vi "main.vi"() -> ()   [LabVIEW 2024]
uses:
  C:/Users/QLM-CCD/Desktop/Pump probe/Kinesis/Thorlabs.MotionControl.Benchtop.BrushlessMotorCLI.dll
  Kinesis/Thorlabs.MotionControl.Benchtop.BrushlessMotorCLI.dll
  <vilib>/Utility/file.llb/Read Delimited Spreadsheet (DBL).vi
  <vilib>/Utility/file.llb/Write Delimited Spreadsheet (DBL).vi
  C:/Users/QLM-CCD/Desktop/Pump probe/Kinesis/Thorlabs.MotionControl.Controls.dll
  Kinesis/Thorlabs.MotionControl.Controls.dll
  <instrlib>/Thorlabs_MC2000B/Thorlabs_MC2000B.lvlib
panel:
  out "return value":string[](array[string])
  out "pp_sig_avg":dbl[](array[numeric])
  out "pp_sig_sum":dbl[](array[numeric])
  in  "Tab Control":enum32{"main", "advanced", "documents"}(tab)
  out "is_measure":bool
  in  "measure_rounds":i16=1 caption="X"
  out "current_delay":dbl caption="fs" format="%#_5g"
  in  "stop":bool
  out "pump probe signal cont":dbl(graph)
  in  "Save_data_path":path=path "C:/Users/QLM-CCD/Desktop/Pump probe/test/test.txt"
  out "XY Graph":cluster{"Y":dbl[], "Y":dbl[]}[](graph)
  out "measure_progress":u8(slide) scale=0.0..12.0
  in  "measure":bool
  in  "Set zero":bool
  in  "measure_cont":bool
  out "is_measure_cont":bool
  in  "delay_profile":u16(ring) caption="delay profile" items=["test", "test2", "test3"]
  in  "set delay":dbl caption="move"
  in  "Set frequency (Hz)":i32=1000
  out "Chopper Frequency (Hz)":i32 caption="chopper freq."
  in  "set lock-in Integration time":dbl=100.0 caption="integration time"
  in  "delay list":dbl[](array[numeric])
  in  "device position (mm)":dbl
  out "Lock-in Integration time":dbl caption="integration time"
  in  "BenchtopBrushlessControl":refnum<k24>(container)
  in  "stop 2":bool
  in  "save_profile":bool
  in  "profile_name":string caption="delay profile"
  in  "open_doc_SR830":bool
  in  "open_doc_MC2000B":bool
  in  "open_doc_BBD301":bool
  out "pp_sig_sgl":dbl[](array[numeric])
  # "todo: state machine,\nfs-ps switch,, note box, issue report box, change color when delay stage is moveing,  measure background, hide kinesis panel"
  # "#BUG: Start measurement without save file will crash"
  # "pump probe  ver0.1.1  2024.08.02"
  # "Hz"
  # "Hz"
  # "ms"
  # "ms"
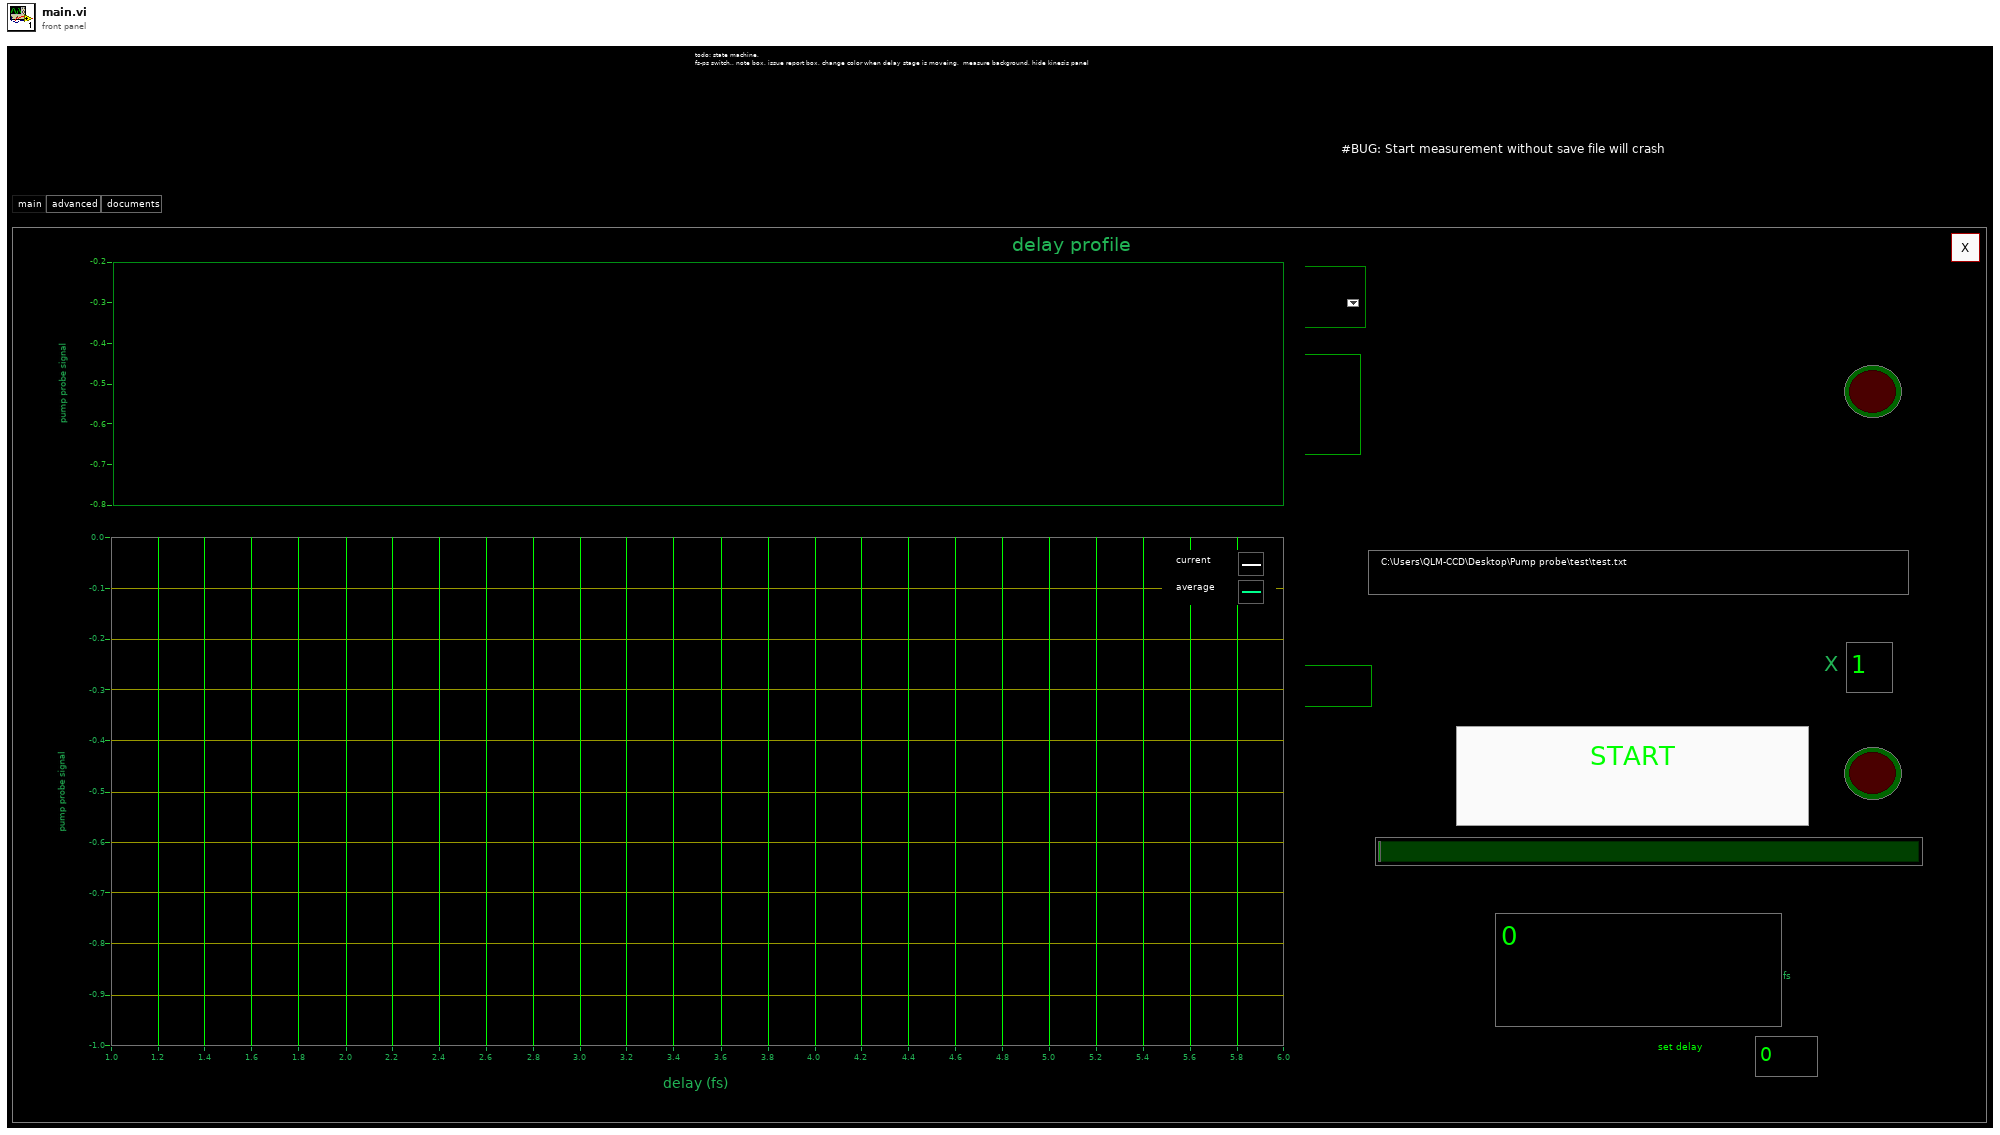
[diagram p1: front panel]
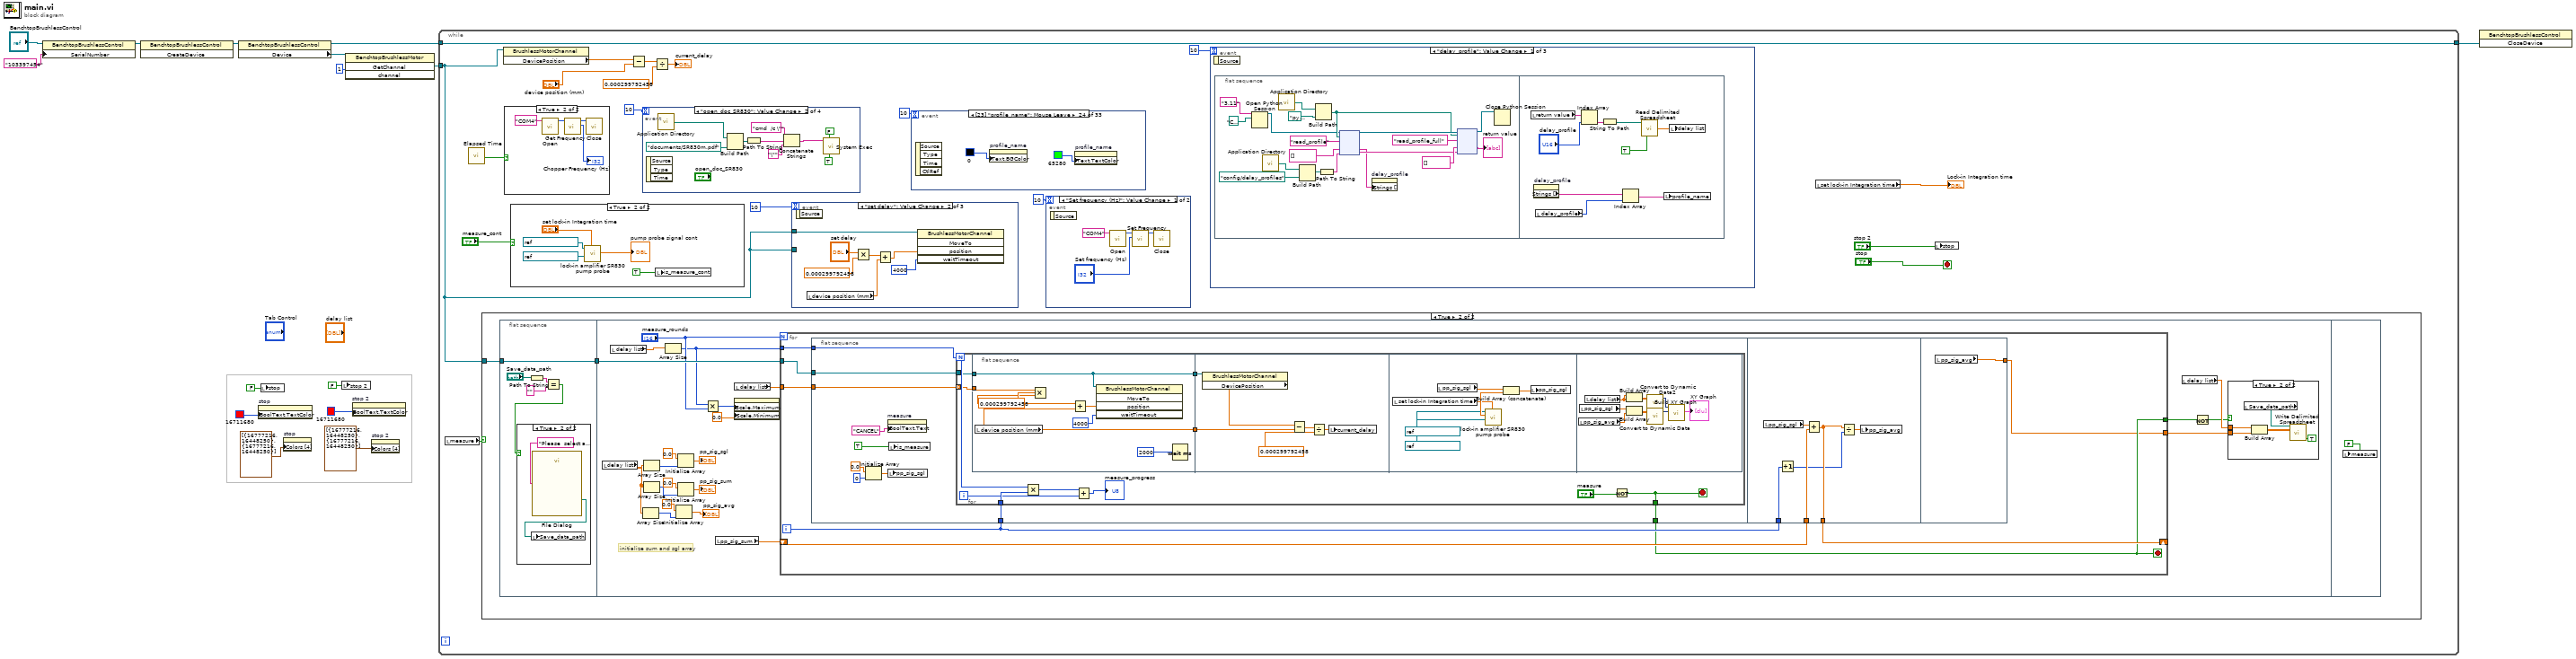
[diagram p0: block diagram]
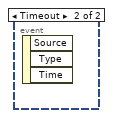
[diagram p2: hidden frame]
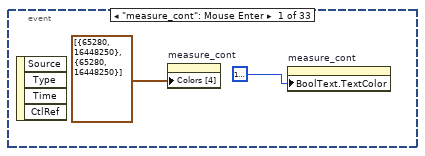
[diagram p3: hidden frame]
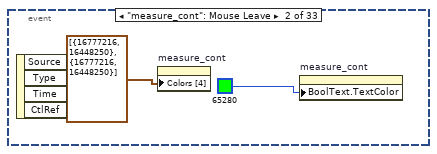
[diagram p4: hidden frame]
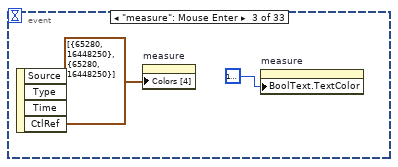
[diagram p5: hidden frame]
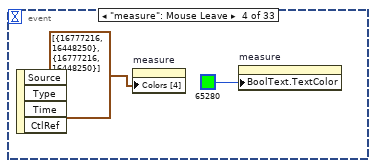
[diagram p6: hidden frame]
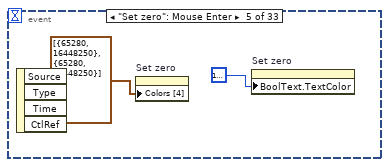
[diagram p7: hidden frame]
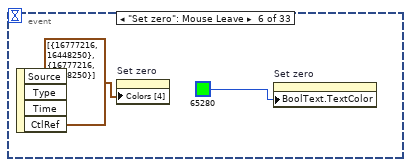
[diagram p8: hidden frame]
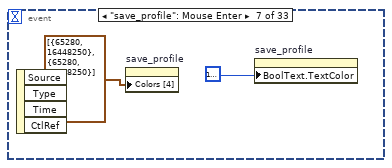
[diagram p9: hidden frame]
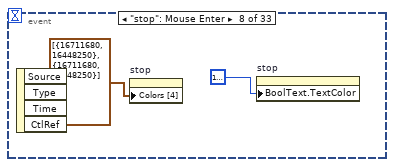
[diagram p10: hidden frame]
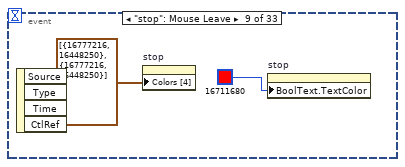
[diagram p11: hidden frame]
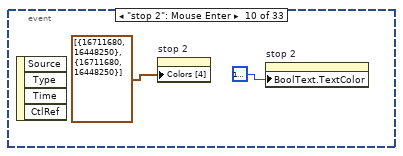
[diagram p12: hidden frame]
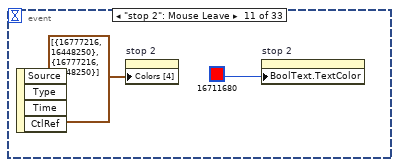
[diagram p13: hidden frame]
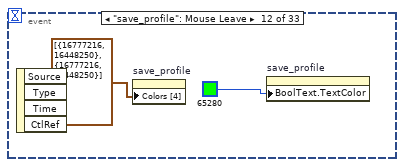
[diagram p14: hidden frame]
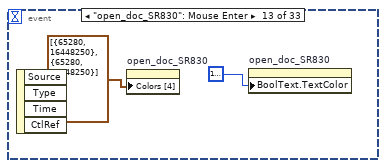
[diagram p15: hidden frame]
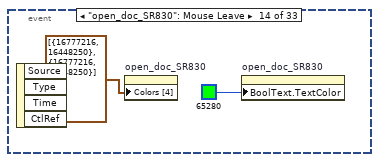
[diagram p16: hidden frame]
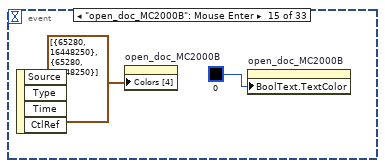
[diagram p17: hidden frame]
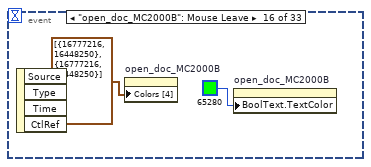
[diagram p18: hidden frame]
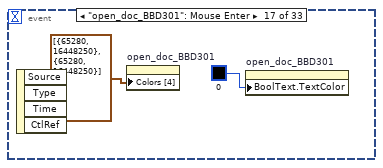
[diagram p19: hidden frame]
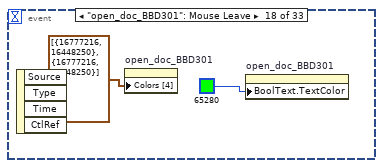
[diagram p20: hidden frame]
diagram:
  n1 = property class="BenchtopBrushlessControl"(reference="BenchtopBrushlessControl", "SerialNumber"="103397454") -> (reference out=w14:refnum<k24>)  [unwired: 1 in, 1 out]
  n2 = invoke class="BenchtopBrushlessControl" method="CreateDevice"(reference=w14) -> (reference out=w13:refnum<k24>)  [unwired: 2 in, 2 out]
  n3 = property class="BenchtopBrushlessControl"(reference=w13) -> (reference out=w11:refnum<k24>, "Device"=w5:refnum<k24>)  [unwired: 1 in, 1 out]
  n4 = property on="stop" class="Bool (strict)"("BoolText.TextColor"=u32 16711680) -> ()  [unwired: 2 in, 2 out]
  n5 = local write "stop"(FALSE ("is_measure")) -> ()
  n6 = property on="stop" class="Bool (strict)"("Colors [4]"=cluster{u32, u32}[] [{16777216, 16448250}, {16777216, 16448250}]) -> ()  [unwired: 2 in, 2 out]
  n7 = local write "stop 2"(FALSE ("is_measure")) -> ()
  n8 = invoke class="BenchtopBrushlessMotor" method="GetChannel"(reference=w5, "channel"=i16 1) -> ("GetChannel"=w8:refnum<k24>)  [unwired: 2 in, 3 out]
  n9 = property on="stop 2" class="Bool (strict)"("BoolText.TextColor"=u32 16711680) -> ()  [unwired: 2 in, 2 out]
  n10 = property on="stop 2" class="Bool (strict)"("Colors [4]"=cluster{u32, u32}[] [{16777216, 16448250}, {16777216, 16448250}]) -> ()  [unwired: 2 in, 2 out]
  n11 = while {
    tunnel: w11 -> [w33]
    tunnel: [w33] -> w10
    tunnel: w8 -> [w16]
    stop <- "stop" stop-if-true
    n12 = local read "measure"() -> (w22:bool)
    n13 = call "Elapsed Time"() -> ("Time has Elapsed"=w27:bool)  [unwired: 12 in, 7 out]
    n14 = case shown="True" w22 {
      tunnel: w16 -> [_ w106]
      frame False {
        n15 = local write "measure_progress"(u8 0 ("measure_progress")) -> ()
        n16 = property on="measure" class="Bool (strict)"("BoolText.Text"="START" ("Boolean Text.Text")) -> ()  [unwired: 2 in, 2 out]
        "is_measure" <- FALSE ("is_measure")
      }
      frame True {
        n17 = flat-sequence {
          tunnel: w106 -> [w111]
          tunnel: [w111] -> w105
          tunnel: w105 -> [w125]
          frame #0 {
            n18 = Path To String(path="Save_data_path") -> (string=w110:string)
            n19 = Equal?(x=w110, y="") -> (x = y?=w107:bool)
            n20 = case shown="True" w107 {
              frame False {
              }
              frame True {
                n21 = call "File Dialog"("prompt"="Please  select a file to save your data") -> ("selected path"=w112:path)  [unwired: 11 in, 3 out]
                n22 = local write "Save_data_path"(w112) -> ()
              }
            }
          }
          frame #1 {
            # "initialize sum and sgl array"
            n23 = local read "delay list"() -> (w122:dbl[])
            n24 = local read "delay list"() -> (w134:dbl[])
            n25 = Array Size(array=w122) -> (size(s)=w123:i32)
            n26 = Array Size(array=w122) -> (size(s)=w131:i32)
            n27 = Array Size(array=w122) -> (size(s)=w129:i32)
            n28 = Array Size(array=w134) -> (size(s)=w116:i32)
            n29 = Initialize Array(0.0 ("element"), w123) -> (→"pp_sig_avg":dbl[])
            n30 = Initialize Array(0.0 ("element"), w131) -> (→"pp_sig_sgl":dbl[])
            n31 = Initialize Array(0.0 ("element"), w129) -> (→"pp_sig_sum":dbl[])
            n32 = Multiply(x=w116, y="measure_rounds") -> (x*y=w135:i32)
            n33 = local read "pp_sig_sum"() -> (w128:dbl[])
            n34 = local read "delay list"() -> (w118:dbl[])
            n35 = property on="measure_progress" class="Slide (strict)"("Scale.Maximum"=w135, "Scale.Minimum"=0.0 ("Scale.Range:Minimum")) -> ()  [unwired: 2 in, 2 out]
            n36 = for {
              N: "measure_rounds" -> [_]
              tunnel: w125 -> [w138]
              shift-right: [w143] -> _
              shift-left: w128 -> [w142]
              tunnel: w118 -> [w140]
              tunnel: [w139] -> w117
              tunnel: w116 -> [w137]
              tunnel: [w136] -> w114
              i -> [w141]
              stop <- w139 stop-if-true
              n37 = flat-sequence {
                tunnel: w141 -> [w153]
                tunnel: [w152] -> w139
                tunnel: w140 -> [w151]
                tunnel: w138 -> [w148]
                tunnel: w137 -> [w147]
                tunnel: w141 -> [w194]
                tunnel: [w197] -> w143
                tunnel: w142 -> [w196]
                tunnel: [w199] -> w136
                frame #0 {
                  n38 = Initialize Array(0.0 ("element"), 0 ("dimension size")) -> (w146:dbl[])
                  n39 = property on="measure" class="Bool (strict)"("BoolText.Text"="CANCEL" ("Boolean Text.Text")) -> ()  [unwired: 2 in, 2 out]
                  n40 = local write "pp_sig_sgl"(w146) -> ()
                  n41 = local write "is_measure"(TRUE ("is_measure")) -> ()
                  n42 = for {
                    N: w147 -> [w160]
                    tunnel: [w159] -> w152
                    tunnel: w153 -> [w161]
                    tunnel: w151 -> [w156] mode=indexing
                    tunnel: w148 -> [w155]
                    i -> [w157]
                    stop <- w159 stop-if-true
                    n43 = flat-sequence {
                      tunnel: [w169] -> w164
                      tunnel: w156 -> [w167]
                      tunnel: w155 -> [w165]
                      tunnel: [w165] -> w154
                      tunnel: w164 -> [w177]
                      tunnel: w154 -> [w173]
                      frame #0 {
                        n44 = local read "device position (mm)"() -> (w169:dbl)
                        n45 = Multiply(x=w167, y=0.000299792458) -> (x*y=w172:dbl)
                        n46 = Add(x=w172, y=w169) -> (x+y=w170:dbl)
                        n47 = invoke class="BrushlessMotorChannel" method="MoveTo"(reference=w165, "position"=w170, "waitTimeout"=4000) -> ()  [unwired: 2 in, 5 out]
                        n48 = Wait (ms)(milliseconds to wait=u32 2000) -> ()  [unwired: 1 out]
                      }
                      frame #1 {
                        n49 = property class="BrushlessMotorChannel"(reference=w173) -> ("DevicePosition"=w174:dbl)  [unwired: 1 in, 2 out]
                        n50 = Subtract(x=w174, y=w177) -> (x-y=w178:dbl)
                        n51 = Divide(x=w178, y=0.000299792458) -> (x/y=w176:dbl)
                        n52 = local write "current_delay"(w176) -> ()
                      }
                      frame #2 {
                        n53 = local read "set lock-in Integration time"() -> (w181:dbl)
                        n54 = local read "pp_sig_sgl"() -> (w180:dbl[])
                        n55 = call "lock-in amplifier SR830 pump probe.vi"("Integration time (ms)"=w181, "Connection 2"=refnum<visa-resource-name> "GPIB0::5::INSTR", "Connection"=refnum<visa-resource-name> "GPIB1::2::INSTR") -> ("pump probe signal"=w183:dbl)  [unwired: 8 in]
                        n56 = Build Array (concatenate)(w180, w183) -> (w179:dbl[])
                        n57 = local write "pp_sig_sgl"(w179) -> ()
                      }
                      frame #3 {
                        n58 = local read "pp_sig_avg"() -> (w187:dbl[])
                        n59 = local read "pp_sig_sgl"() -> (w185:dbl[])
                        n60 = local read "delay list"() -> (w190:dbl[])
                        n61 = Build Array(w190, w190) -> (w189:dbl[][])
                        n62 = Build Array(w185, w187) -> (w191:dbl[][])
                        n63 = call "Convert to Dynamic Data2"("2D Array"=w189) -> ("Dynamic Data Type"=w188:dynamicdata)  [unwired: 3 in]
                        n64 = call "Convert to Dynamic Data"("2D Array"=w191) -> ("Dynamic Data Type"=w192:dynamicdata)  [unwired: 3 in]
                        n65 = call "Build XY Graph"("Y Input"=w192, "X Input"=w188) -> ("XY Graph"=→"XY Graph":cluster{"X":dbl[], "Y":dbl[]}[])  [unwired: 8 in, 1 out]
                      }
                    }
                    n66 = Multiply(x=w160, y=w161) -> (x*y=w158:i32)
                    n67 = Add(x=w158, y=w157) -> (x+y=→"measure_progress":i32)
                    n68 = Not(x="measure") -> (.not. x?=w159:bool)
                  }
                }
                frame #1 {
                  n69 = local read "pp_sig_sgl"() -> (w198:dbl[])
                  n70 = Increment(x=w194) -> (x+1=w193:i32)
                  n71 = Add(x=w198, y=w196) -> (x+y=w197:dbl[])
                  n72 = Divide(x=w197, y=w193) -> (x/y=w195:dbl[])
                  n73 = local write "pp_sig_avg"(w195) -> ()
                }
                frame #2 {
                  n74 = local read "pp_sig_avg"() -> (w199:dbl[])
                }
              }
            }
            n75 = local read "delay list"() -> (w133:dbl[])
            n76 = Not(x=w117) -> (.not. x?=w115:bool)
            n77 = case shown="True" w115 {
              tunnel: w133 -> [_ w202]
              tunnel: w114 -> [_ w200]
              frame False {
              }
              frame True {
                n78 = local read "Save_data_path"() -> (w201:path)
                n79 = Build Array(w202, w200) -> (w204:dbl[][])
                n80 = call-poly <vilib>:"Write Delimited Spreadsheet.vi"("file path (dialog if empty)"=w201, "2D data"=w204, "transpose? (no:F)"=TRUE) -> ()  [unwired: 11 in, 2 out]
              }
            }
          }
          frame #2 {
            n81 = local write "measure"(FALSE ("measure")) -> ()
          }
        }
      }
    }
    n82 = property class="BrushlessMotorChannel"(reference=w16) -> ("DevicePosition"=w31:dbl)  [unwired: 1 in, 2 out]
    n83 = case shown="True" w27 {
      frame False {
      }
      frame True {
        n84 = call <instrlib>:"Open.vi"("Serial Port"="COM4") -> ("Handle out"=w278:i32)  [unwired: 8 in, 2 out]
        n85 = call <instrlib>:"Get Frequency.vi"("Handle in"=w278) -> ("Frequency (Hz)"=→"Chopper Frequency (Hz)":i32, "Handle out"=w277:i32)  [unwired: 8 in, 1 out]
        n86 = call <instrlib>:"Close.vi"("hdl"=w277) -> ()  [unwired: 10 in, 1 out]
      }
    }
    n87 = case shown="True" "measure_cont" {
      frame False {
        "is_measure_cont" <- FALSE ("is_measure_cont")
      }
      frame True {
        n88 = call "lock-in amplifier SR830 pump probe.vi"("Integration time (ms)"="set lock-in Integration time", "Connection 2"=refnum<visa-resource-name> "GPIB0::5::INSTR", "Connection"=refnum<visa-resource-name> "GPIB1::2::INSTR") -> ("pump probe signal"=→"pump probe signal cont":dbl)  [unwired: 8 in]
        n89 = local write "is_measure_cont"(TRUE ("is_measure_cont")) -> ()
      }
    }
    n90 = Subtract(x=w31, y="device position (mm)") -> (x-y=w30:dbl)
    n91 = event shown="[1] \"open_doc_SR830\": Value Change" {
      selector: _ -> [_ _ _ _]
      dyn-events: _ -> [_ _ _ _]
      timeout: 10 -> [_ _ _ _]
      event Timeout {
        n92 = event-data() -> ()  [unwired: 1 in, 3 out]
      }
      event "open_doc_SR830": Value Change {
        n93 = event-data() -> ()  [unwired: 1 in, 3 out]
        n94 = call <vilib>:"Application Directory.vi"() -> ("Application Directory"=w245:path)
        n95 = Build Path(base path=w245, name or relative path=path "documents/SR830m.pdf") -> (appended path=w246:path)
        n96 = Path To String(path=w246) -> (string=w244:string)
        n97 = Concatenate Strings("cmd  /c \"" ("string"), w244, "\"" ("string")) -> (w250:string)
        n98 = call <vilib>:"System Exec.vi"("run minimized? (F)"=TRUE, "wait until completion? (T)"=FALSE, "command line"=w250) -> ()  [unwired: 5 in, 4 out]
      }
      event "open_doc_MC2000B": Value Change {
        n99 = event-data() -> ()  [unwired: 1 in, 3 out]
        n100 = call <vilib>:"Application Directory.vi"() -> ("Application Directory"=w254:path)
        n101 = Build Path(base path=w254, name or relative path=path "documents/MC2000B-Manual.pdf") -> (appended path=w255:path)
        n102 = Path To String(path=w255) -> (string=w252:string)
        n103 = Concatenate Strings("cmd  /c \"" ("string"), w252, "\"" ("string")) -> (w259:string)
        n104 = call <vilib>:"System Exec.vi"("run minimized? (F)"=TRUE, "wait until completion? (T)"=FALSE, "command line"=w259) -> ()  [unwired: 5 in, 4 out]
      }
      event "open_doc_BBD301": Value Change {
        n105 = event-data() -> ()  [unwired: 1 in, 1 out]
        n106 = call <vilib>:"Application Directory.vi"() -> ("Application Directory"=w263:path)
        n107 = Build Path(base path=w263, name or relative path=path "documents/BBD301-KinesisManual.pdf") -> (appended path=w264:path)
        n108 = Path To String(path=w264) -> (string=w261:string)
        n109 = Concatenate Strings("cmd  /c \"" ("string"), w261, "\"" ("string")) -> (w268:string)
        n110 = call <vilib>:"System Exec.vi"("run minimized? (F)"=TRUE, "wait until completion? (T)"=FALSE, "command line"=w268) -> ()  [unwired: 5 in, 4 out]
      }
    }
    n111 = Divide(x=w30, y=0.000299792458) -> (x/y=→"current_delay":dbl)
    n112 = event shown="[1] \"set delay\": Value Change" {
      selector: _ -> [_ _ _]
      dyn-events: _ -> [_ _ _]
      timeout: 10 -> [_ _ _]
      tunnel: w16 -> [w281 _ _]
      tunnel: w16 -> [_ w283 _]
      event "Set zero": Value Change {
        n113 = event-data() -> ()  [unwired: 1 in, 1 out]
        n114 = property class="BrushlessMotorChannel"(reference=w281) -> ("DevicePosition"=w280:dbl)  [unwired: 1 in, 2 out]
        n115 = local write "device position (mm)"(w280) -> ()
      }
      event "set delay": Value Change {
        n116 = event-data() -> ()  [unwired: 1 in, 1 out]
        n117 = local read "device position (mm)"() -> (w282:dbl)
        n118 = Multiply(x="set delay", y=0.000299792458) -> (x*y=w285:dbl)
        n119 = Add(x=w285, y=w282) -> (x+y=w284:dbl)
        n120 = invoke class="BrushlessMotorChannel" method="MoveTo"(reference=w283, "position"=w284, "waitTimeout"=4000) -> ()  [unwired: 2 in, 5 out]
      }
      event Timeout {
        n121 = event-data() -> ()  [unwired: 1 in, 3 out]
      }
    }
    n122 = event shown="[23] \"profile_name\": Mouse Leave" {
      selector: _ -> [_ _ _ _ _ _ _ _ _ _ _ _ _ _ _ _ _ _ _ _ _ _ _ _ _ _ _ _ _ _ _ _ _]
      dyn-events: _ -> [_ _ _ _ _ _ _ _ _ _ _ _ _ _ _ _ _ _ _ _ _ _ _ _ _ _ _ _ _ _ _ _ _]
      timeout: 10 -> [_ _ _ _ _ _ _ _ _ _ _ _ _ _ _ _ _ _ _ _ _ _ _ _ _ _ _ _ _ _ _ _ _]
      event "measure_cont": Mouse Enter {
        n123 = event-data() -> ()  [unwired: 1 in, 4 out]
        n124 = property on="measure_cont" class="Bool (strict)"("Colors [4]"=cluster{u32, u32}[] [{65280, 16448250}, {65280, 16448250}]) -> ()  [unwired: 2 in, 2 out]
        n125 = property on="measure_cont" class="Bool (strict)"("BoolText.TextColor"=u32 16777222) -> ()  [unwired: 2 in, 2 out]
      }
      event "measure_cont": Mouse Leave {
        n126 = event-data() -> ()  [unwired: 1 in, 4 out]
        n127 = property on="measure_cont" class="Bool (strict)"("Colors [4]"=cluster{u32, u32}[] [{16777216, 16448250}, {16777216, 16448250}]) -> ()  [unwired: 2 in, 2 out]
        n128 = property on="measure_cont" class="Bool (strict)"("BoolText.TextColor"=u32 65280) -> ()  [unwired: 2 in, 2 out]
      }
      event "measure": Mouse Enter {
        n129 = event-data() -> ()  [unwired: 1 in, 4 out]
        n130 = property on="measure" class="Bool (strict)"("Colors [4]"=cluster{u32, u32}[] [{65280, 16448250}, {65280, 16448250}]) -> ()  [unwired: 2 in, 2 out]
        n131 = property on="measure" class="Bool (strict)"("BoolText.TextColor"=u32 16777222) -> ()  [unwired: 2 in, 2 out]
      }
      event "measure": Mouse Leave {
        n132 = event-data() -> ()  [unwired: 1 in, 4 out]
        n133 = property on="measure" class="Bool (strict)"("Colors [4]"=cluster{u32, u32}[] [{16777216, 16448250}, {16777216, 16448250}]) -> ()  [unwired: 2 in, 2 out]
        n134 = property on="measure" class="Bool (strict)"("BoolText.TextColor"=u32 65280) -> ()  [unwired: 2 in, 2 out]
      }
      event "Set zero": Mouse Enter {
        n135 = event-data() -> ()  [unwired: 1 in, 4 out]
        n136 = property on="Set zero" class="Bool"("Colors [4]"=cluster{u32, u32}[] [{65280, 16448250}, {65280, 16448250}]) -> ()  [unwired: 2 in, 2 out]
        n137 = property on="Set zero" class="Bool"("BoolText.TextColor"=u32 16777222) -> ()  [unwired: 2 in, 2 out]
      }
      event "Set zero": Mouse Leave {
        n138 = event-data() -> ()  [unwired: 1 in, 4 out]
        n139 = property on="Set zero" class="Bool"("Colors [4]"=cluster{u32, u32}[] [{16777216, 16448250}, {16777216, 16448250}]) -> ()  [unwired: 2 in, 2 out]
        n140 = property on="Set zero" class="Bool"("BoolText.TextColor"=u32 65280) -> ()  [unwired: 2 in, 2 out]
      }
      event "save_profile": Mouse Enter {
        n141 = event-data() -> ()  [unwired: 1 in, 4 out]
        n142 = property on="save_profile" class="Bool"("Colors [4]"=cluster{u32, u32}[] [{65280, 16448250}, {65280, 16448250}]) -> ()  [unwired: 2 in, 2 out]
        n143 = property on="save_profile" class="Bool"("BoolText.TextColor"=u32 16777222) -> ()  [unwired: 2 in, 2 out]
      }
      event "stop": Mouse Enter {
        n144 = event-data() -> ()  [unwired: 1 in, 4 out]
        n145 = property on="stop" class="Bool (strict)"("Colors [4]"=cluster{u32, u32}[] [{16711680, 16448250}, {16711680, 16448250}]) -> ()  [unwired: 2 in, 2 out]
        n146 = property on="stop" class="Bool (strict)"("BoolText.TextColor"=u32 16777222) -> ()  [unwired: 2 in, 2 out]
      }
      event "stop": Mouse Leave {
        n147 = event-data() -> ()  [unwired: 1 in, 4 out]
        n148 = property on="stop" class="Bool (strict)"("Colors [4]"=cluster{u32, u32}[] [{16777216, 16448250}, {16777216, 16448250}]) -> ()  [unwired: 2 in, 2 out]
        n149 = property on="stop" class="Bool (strict)"("BoolText.TextColor"=u32 16711680) -> ()  [unwired: 2 in, 2 out]
      }
      event "stop 2": Mouse Enter {
        n150 = event-data() -> ()  [unwired: 1 in, 4 out]
        n151 = property on="stop 2" class="Bool (strict)"("Colors [4]"=cluster{u32, u32}[] [{16711680, 16448250}, {16711680, 16448250}]) -> ()  [unwired: 2 in, 2 out]
        n152 = property on="stop 2" class="Bool (strict)"("BoolText.TextColor"=u32 16777222) -> ()  [unwired: 2 in, 2 out]
      }
      event "stop 2": Mouse Leave {
        n153 = event-data() -> ()  [unwired: 1 in, 4 out]
        n154 = property on="stop 2" class="Bool (strict)"("Colors [4]"=cluster{u32, u32}[] [{16777216, 16448250}, {16777216, 16448250}]) -> ()  [unwired: 2 in, 2 out]
        n155 = property on="stop 2" class="Bool (strict)"("BoolText.TextColor"=u32 16711680) -> ()  [unwired: 2 in, 2 out]
      }
      event "save_profile": Mouse Leave {
        n156 = event-data() -> ()  [unwired: 1 in, 4 out]
        n157 = property on="save_profile" class="Bool"("Colors [4]"=cluster{u32, u32}[] [{16777216, 16448250}, {16777216, 16448250}]) -> ()  [unwired: 2 in, 2 out]
        n158 = property on="save_profile" class="Bool"("BoolText.TextColor"=u32 65280) -> ()  [unwired: 2 in, 2 out]
      }
      event "open_doc_SR830": Mouse Enter {
        n159 = event-data() -> ()  [unwired: 1 in, 4 out]
        n160 = property on="open_doc_SR830" class="Bool"("Colors [4]"=cluster{u32, u32}[] [{65280, 16448250}, {65280, 16448250}]) -> ()  [unwired: 2 in, 2 out]
        n161 = property on="open_doc_SR830" class="Bool"("BoolText.TextColor"=u32 16777222) -> ()  [unwired: 2 in, 2 out]
      }
      event "open_doc_SR830": Mouse Leave {
        n162 = event-data() -> ()  [unwired: 1 in, 4 out]
        n163 = property on="open_doc_SR830" class="Bool"("Colors [4]"=cluster{u32, u32}[] [{16777216, 16448250}, {16777216, 16448250}]) -> ()  [unwired: 2 in, 2 out]
        n164 = property on="open_doc_SR830" class="Bool"("BoolText.TextColor"=u32 65280) -> ()  [unwired: 2 in, 2 out]
      }
      event "open_doc_MC2000B": Mouse Enter {
        n165 = event-data() -> ()  [unwired: 1 in, 4 out]
        n166 = property on="open_doc_MC2000B" class="Bool"("Colors [4]"=cluster{u32, u32}[] [{65280, 16448250}, {65280, 16448250}]) -> ()  [unwired: 2 in, 2 out]
        n167 = property on="open_doc_MC2000B" class="Bool"("BoolText.TextColor"=u32 0) -> ()  [unwired: 2 in, 2 out]
      }
      event "open_doc_MC2000B": Mouse Leave {
        n168 = event-data() -> ()  [unwired: 1 in, 4 out]
        n169 = property on="open_doc_MC2000B" class="Bool"("Colors [4]"=cluster{u32, u32}[] [{16777216, 16448250}, {16777216, 16448250}]) -> ()  [unwired: 2 in, 2 out]
        n170 = property on="open_doc_MC2000B" class="Bool"("BoolText.TextColor"=u32 65280) -> ()  [unwired: 2 in, 2 out]
      }
      event "open_doc_BBD301": Mouse Enter {
        n171 = event-data() -> ()  [unwired: 1 in, 4 out]
        n172 = property on="open_doc_BBD301" class="Bool"("Colors [4]"=cluster{u32, u32}[] [{65280, 16448250}, {65280, 16448250}]) -> ()  [unwired: 2 in, 2 out]
        n173 = property on="open_doc_BBD301" class="Bool"("BoolText.TextColor"=u32 0) -> ()  [unwired: 2 in, 2 out]
      }
      event "open_doc_BBD301": Mouse Leave {
        n174 = event-data() -> ()  [unwired: 1 in, 4 out]
        n175 = property on="open_doc_BBD301" class="Bool"("Colors [4]"=cluster{u32, u32}[] [{16777216, 16448250}, {16777216, 16448250}]) -> ()  [unwired: 2 in, 2 out]
        n176 = property on="open_doc_BBD301" class="Bool"("BoolText.TextColor"=u32 65280) -> ()  [unwired: 2 in, 2 out]
      }
      event "Set frequency (Hz)": Mouse Enter {
        n177 = event-data() -> ()  [unwired: 1 in, 4 out]
        n178 = property on="Set frequency (Hz)" class="DigNum (strict)"("NumText.BGColor"=u32 65280) -> ()  [unwired: 2 in, 2 out]
        n179 = property on="Set frequency (Hz)" class="DigNum (strict)"("NumText.TextColor"=u32 0) -> ()  [unwired: 2 in, 2 out]
      }
      event "Set frequency (Hz)": Mouse Leave {
        n180 = event-data() -> ()  [unwired: 1 in, 4 out]
        n181 = property on="Set frequency (Hz)" class="DigNum (strict)"("NumText.BGColor"=u32 0) -> ()  [unwired: 2 in, 2 out]
        n182 = property on="Set frequency (Hz)" class="DigNum (strict)"("NumText.TextColor"=u32 65280) -> ()  [unwired: 2 in, 2 out]
      }
      event "set lock-in Integration time": Mouse Enter {
        n183 = event-data() -> ()  [unwired: 1 in, 4 out]
        n184 = property on="set lock-in Integration time" class="DigNum (strict)"("NumText.BGColor"=u32 65280) -> ()  [unwired: 2 in, 2 out]
        n185 = property on="set lock-in Integration time" class="DigNum (strict)"("NumText.TextColor"=u32 0) -> ()  [unwired: 2 in, 2 out]
      }
      event "set lock-in Integration time": Mouse Leave {
        n186 = event-data() -> ()  [unwired: 1 in, 4 out]
        n187 = property on="set lock-in Integration time" class="DigNum (strict)"("NumText.BGColor"=u32 0) -> ()  [unwired: 2 in, 2 out]
        n188 = property on="set lock-in Integration time" class="DigNum (strict)"("NumText.TextColor"=u32 65280) -> ()  [unwired: 2 in, 2 out]
      }
      event "profile_name": Mouse Enter {
        n189 = event-data() -> ()  [unwired: 1 in, 4 out]
        n190 = property on="profile_name" class="Str"("Text.BGColor"=u32 65280) -> ()  [unwired: 2 in, 2 out]
        n191 = property on="profile_name" class="Str"("Text.TextColor"=u32 0) -> ()  [unwired: 2 in, 2 out]
      }
      event "profile_name": Mouse Leave {
        n192 = event-data() -> ()  [unwired: 1 in, 4 out]
        n193 = property on="profile_name" class="Str"("Text.BGColor"=u32 0) -> ()  [unwired: 2 in, 2 out]
        n194 = property on="profile_name" class="Str"("Text.TextColor"=u32 65280) -> ()  [unwired: 2 in, 2 out]
      }
      event "delay_profile": Mouse Enter {
        n195 = event-data() -> ()  [unwired: 1 in, 4 out]
        n196 = property on="delay_profile" class="Ring (strict)"("RingText.BGColor"=u32 65280) -> ()  [unwired: 2 in, 2 out]
        n197 = property on="delay_profile" class="Ring (strict)"("RingText.TextColor"=u32 0) -> ()  [unwired: 2 in, 2 out]
      }
      event "delay_profile": Mouse Leave {
        n198 = event-data() -> ()  [unwired: 1 in, 4 out]
        n199 = property on="delay_profile" class="Ring (strict)"("RingText.BGColor"=u32 16777216) -> ()  [unwired: 2 in, 2 out]
        n200 = property on="delay_profile" class="Ring (strict)"("RingText.TextColor"=u32 65280) -> ()  [unwired: 2 in, 2 out]
      }
      event "set delay": Mouse Enter {
        n201 = event-data() -> ()  [unwired: 1 in, 4 out]
        n202 = property on="set delay" class="DigNum (strict)"("NumText.BGColor"=u32 65280) -> ()  [unwired: 2 in, 2 out]
        n203 = property on="set delay" class="DigNum (strict)"("NumText.TextColor"=u32 0) -> ()  [unwired: 2 in, 2 out]
      }
      event "set delay": Mouse Leave {
        n204 = event-data() -> ()  [unwired: 1 in, 4 out]
        n205 = property on="set delay" class="DigNum (strict)"("NumText.BGColor"=u32 16777222) -> ()  [unwired: 2 in, 2 out]
        n206 = property on="set delay" class="DigNum (strict)"("NumText.TextColor"=u32 65280) -> ()  [unwired: 2 in, 2 out]
      }
      event "measure_rounds": Mouse Enter {
        n207 = event-data() -> ()  [unwired: 1 in, 4 out]
        n208 = property on="measure_rounds" class="DigNum (strict)"("NumText.BGColor"=u32 65280) -> ()  [unwired: 2 in, 2 out]
        n209 = property on="measure_rounds" class="DigNum (strict)"("NumText.TextColor"=u32 0) -> ()  [unwired: 2 in, 2 out]
      }
      event "measure_rounds": Mouse Leave {
        n210 = event-data() -> ()  [unwired: 1 in, 4 out]
        n211 = property on="measure_rounds" class="DigNum (strict)"("NumText.BGColor"=u32 0) -> ()  [unwired: 2 in, 2 out]
        n212 = property on="measure_rounds" class="DigNum (strict)"("NumText.TextColor"=u32 65280) -> ()  [unwired: 2 in, 2 out]
      }
      event "Save_data_path": Mouse Enter {
        n213 = event-data() -> ()  [unwired: 1 in, 4 out]
        n214 = property on="Save_data_path" class="Path"("Text.BGColor"=u32 16777226) -> ()  [unwired: 2 in, 2 out]
        n215 = property on="Save_data_path" class="Path"("Text.TextColor"=u32 0) -> ()  [unwired: 2 in, 2 out]
      }
      event "Save_data_path": Mouse Leave {
        n216 = event-data() -> ()  [unwired: 1 in, 4 out]
        n217 = property on="Save_data_path" class="Path"("Text.BGColor"=u32 0) -> ()  [unwired: 2 in, 2 out]
        n218 = property on="Save_data_path" class="Path"("Text.TextColor"=u32 16777226) -> ()  [unwired: 2 in, 2 out]
      }
      event Timeout {
        n219 = event-data() -> ()  [unwired: 1 in, 3 out]
      }
    }
    n220 = event shown="[0] \"Set frequency (Hz)\": Value Change" {
      selector: _ -> [_ _]
      dyn-events: _ -> [_ _]
      timeout: 10 -> [_ _]
      event "Set frequency (Hz)": Value Change {
        n221 = event-data() -> ()  [unwired: 1 in, 1 out]
        n222 = call <instrlib>:"Open.vi"("Serial Port"="COM4") -> ("Handle out"=w35:i32)  [unwired: 8 in, 2 out]
        n223 = call <instrlib>:"Set Frequency.vi"("Frequency (Hz)"="Set frequency (Hz)", "Handle in"=w35) -> ("Handle out"=w37:i32)  [unwired: 8 in, 1 out]
        n224 = call <instrlib>:"Close.vi"("hdl"=w37) -> ()  [unwired: 10 in, 1 out]
      }
      event Timeout {
        n225 = event-data() -> ()  [unwired: 1 in, 3 out]
      }
    }
    n226 = event shown="[0] \"delay_profile\": Value Change" {
      selector: _ -> [_ _ _]
      dyn-events: _ -> [_ _ _]
      timeout: 10 -> [_ _ _]
      event "delay_profile": Value Change {
        n227 = event-data() -> ()  [unwired: 1 in, 1 out]
        n228 = flat-sequence {
          frame #0 {
            n229 = Open Python Session(python version="3.11" ("Python version"), python path=path "C:/Users/QLM-CCD/AppData/Local/Programs/Python/Python311-32/pythonw.exe" ("Python path")) -> (session out=w206:refnum<k35>)  [unwired: 1 in, 1 out]
            n230 = call <vilib>:"Application Directory.vi"() -> ("Application Directory"=w220:path)
            n231 = call <vilib>:"Application Directory.vi"() -> ("Application Directory"=w224:path)
            n232 = Build Path(base path=w220, name or relative path=path "config/delay_profiles") -> (appended path=w218:path)
            n233 = Build Path(base path=w224, name or relative path=path "python/functions.py") -> (appended path=w214:path)
            n234 = Path To String(path=w218) -> (string=w217:string)
            n235 = node(w206, w214, "read_profile" ("function name"), string[] [], w217) -> (w216:refnum<k35>, w209:string[], w211:string)  [unwired: 1 in, 3 out]
            n236 = property on="delay_profile" class="Ring (strict)"("Strings []"=w209) -> ()  [unwired: 2 in, 2 out]
            n237 = node(w216, w214, "read_profile_full" ("function name"), string[] [], w211) -> (w215:refnum<k35>, →"return value":string[])  [unwired: 2 in, 3 out]
            n238 = Close Python Session(session in=w215) -> ()  [unwired: 1 in, 1 out]
          }
          frame #1 {
            n239 = local read "return value"() -> (w227:string[])
            n240 = property on="delay_profile" class="Ring (strict)"() -> ("Strings []"=w232:string[])  [unwired: 2 in, 2 out]
            n241 = local read "delay_profile"() -> (w231:u16)
            n242 = Index Array(array=w227, index="delay_profile") -> (element=w228:string)
            n243 = String To Path(string=w228) -> (path=w233:path)
            n244 = Index Array(array=w232, index=w231) -> (element=w230:string)
            n245 = call-poly <vilib>:"Read Delimited Spreadsheet.vi"("file path (dialog if empty)"=w233, "transpose? (F)"=TRUE) -> ("first row"=w229:dbl[])  [unwired: 8 in, 5 out]
            n246 = local write "profile_name"(w230) -> ()
            n247 = local write "delay list"(w229) -> ()
          }
        }
      }
      event "save_profile": Value Change {
        n248 = event-data() -> ()  [unwired: 1 in, 6 out]
        n249 = Concatenate Strings("config\\delay_profiles\\" ("string"), "profile_name", ".txt" ("string")) -> (w239:string)
        n250 = call <vilib>:"Application Directory.vi"() -> ("Application Directory"=w238:path)
        n251 = String To Path(string=w239) -> (path=w237:path)
        n252 = Build Path(base path=w238, name or relative path=w237) -> (appended path=w236:path)
        n253 = local read "delay list"() -> (w234:dbl[])
        n254 = call-poly <vilib>:"Write Delimited Spreadsheet.vi"("file path (dialog if empty)"=w236, "1D data"=w234, "transpose? (no:F)"=TRUE) -> ()  [unwired: 11 in, 2 out]
      }
      event Timeout {
        n255 = event-data() -> ()  [unwired: 1 in, 3 out]
      }
    }
    n256 = local read "set lock-in Integration time"() -> (→"Lock-in Integration time":dbl)
    n257 = local write "stop"("stop 2") -> ()
  }
  n258 = invoke class="BenchtopBrushlessControl" method="CloseDevice"(reference=w10) -> ()  [unwired: 2 in, 3 out]
